vi "index-bit.vi"(10 "index":i32, 11 "array":u8[](array[numeric])) -> (0 "bit3":bool, 1 "bit6":bool, 2 "bit2":bool, 3 "bit7":bool, 4 "bit4":bool, 5 "bit1":bool, 6 "bit5":bool, 7 "bit0":bool)   [LabVIEW 2012]
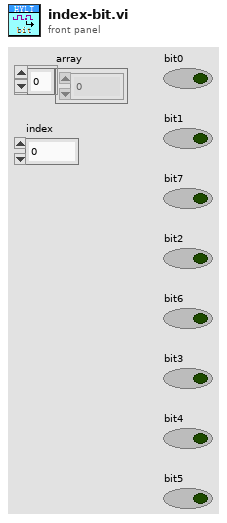
[diagram p1: front panel]
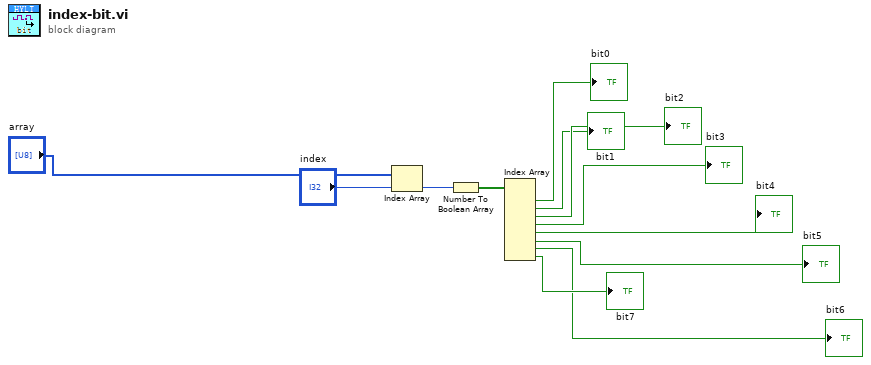
[diagram p0: block diagram]
diagram:
  n1 = Index Array(array="array", index="index") -> (element=w3:u8)
  n2 = Number To Boolean Array(number=w3) -> (Boolean array=w4:bool[])
  n3 = Index Array(array=w4) -> (element #1=→"bit0":bool, element #2=→"bit1":bool, element #3=→"bit2":bool, element #4=→"bit3":bool, element #5=→"bit4":bool, element #6=→"bit5":bool, element #7=→"bit6":bool, element #8=→"bit7":bool)  [unwired: 8 in]
